vi "Delete.vi"(11 "Msg Input in":refnum<class "Msg Input.lvclass">) -> ()   [LabVIEW 2020, in "jettl.lvlib" / "Msg Input.lvclass"]
uses:
  Msg Input.lvclass
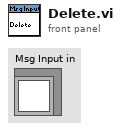
[diagram p1: front panel]
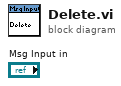
[diagram p0: block diagram]
diagram:
